vi "Setup UI.vi"(8 "error in (no error)":errorcluster, 10 "?":bool, 11 "LCD Reader in":refnum<class "LCD Reader.lvclass">) -> (0 "error out":errorcluster, 3 "LCD Reader out":refnum<class "LCD Reader.lvclass">)   [LabVIEW 2012, in "LCD Reader.lvclass"]
doc: "Setup UI constructs an object -- populates its member data -- from a front panel the user can see. The VI should be as simple as possible so that a UI loop can poll it continuously for updates. \n\nThe VI is designed to be used as a subPanel within another VI. Wire true to \"Set UI to input\" only on the first call, just after inserting this VI into a subPanel, to populate its controls with the class's current values.\n\nSetup UI is distinct from the class constructor. Class constructors are not polymorphic, yet configure dialogs need to configure objects without knowing their type -- and polymorphism is the necessary solution. Thus, Setup UI is a polymorphic class constructor. This continously polled \"Setup UI\" concept is a kludge: a better idea would be an XControl, but those require a steeper learning curve."
uses:
  LCD Reader.lvclass
  LCD Reader.lvclass/LCD Reader.ctl
  Reader/Reader.lvclass
  Instruments/LCD/LCD Retarder.lvclass
panel:
  in  "?":bool
  in  "LCD 1/4 Wave Retardance":dbl[unit]
  # "Set Retardance"
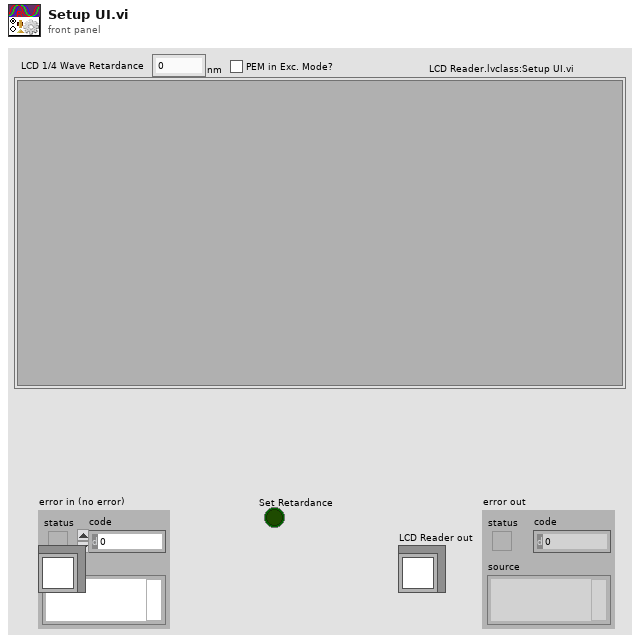
[diagram p1: front panel]
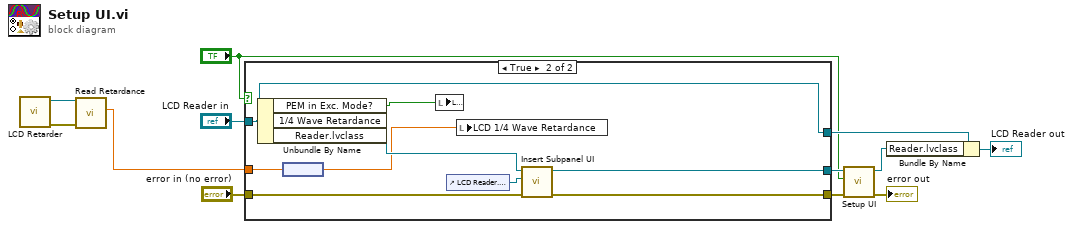
[diagram p0: block diagram]
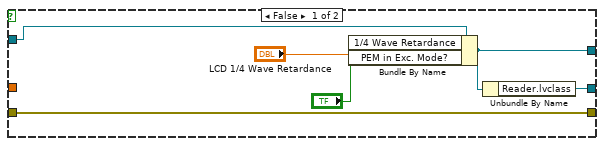
[diagram p2: hidden frame]
diagram:
  n1 = call "LCD Retarder.vi"() -> ("errorOUT"=w2:errorcluster, "LCD out"=w3:refnum<class "LCD Retarder.lvclass">)  [unwired: 10 in]
  n2 = call "Read Retardance.vi"("errorIN"=w2, "LCD in"=w3) -> ("Retardance out"=w1:dbl)  [unwired: 7 in, 2 out]
  n3 = case shown="True" "?" {
    tunnel: "error in (no error)" -> [w18 w27]
    tunnel: [w18 w26] -> w6
    tunnel: "LCD Reader in" -> [w17 w21]
    tunnel: [w14 w21] -> w10
    tunnel: [w13 w22] -> w7
    tunnel: w1 -> [_ w20]
    frame False {
      n4 = Bundle By Name(cluster=w17, "1/4 Wave Retardance"="LCD 1/4 Wave Retardance", "PEM in Exc. Mode?"="?") -> (w14:refnum<class "LCD Reader.lvclass">)
      n5 = Unbundle By Name(w14) -> ("Reader.lvclass"=w13:refnum<class "Reader.lvclass">)
    }
    frame True {
      n6 = Unbundle By Name(w21) -> ("PEM in Exc. Mode?"=w25:bool, "Reader.lvclass"=w24:refnum<class "Reader.lvclass">)  [unwired: 1 out]
      n7 = node(w20) -> (w19:dbl[unit])
      n8 = local write item#6(w25) -> ()
      n9 = control-ref of="LCD Reader.lvclass:Setup UI.vi"() -> (w23:refnum<vi>)
      n10 = local write "LCD 1/4 Wave Retardance"(w19) -> ()
      n11 = call "Insert Subpanel UI.vi"("error in (no error)"=w27, "Subpanel in"=w23, "LabVIEW Object"=w24) -> ("error out"=w26:errorcluster, "LabVIEW Object out"=w22:refnum<class "Reader.lvclass">)  [unwired: 7 out]
    }
  }
  n12 = call-dynamic "Setup UI.vi"("error in (no error)"=w6, "Set UI to input? (F)"="?", "Reader in"=w7) -> ("error out"=→"error out":errorcluster, "Reader out"=w8:refnum<class "Reader.lvclass">)  [unwired: 7 out]
  n13 = Bundle By Name(cluster=w10, "Reader.lvclass"=w8) -> (→"LCD Reader out":refnum<class "LCD Reader.lvclass">)
